vi "SetFunctionClass.vi"(8 "error in (no error)":errorcluster, 10 "FunctionClass":variant, 11 "AnalysisPluginsBase in":refnum<class "AnalysisPluginsBase.lvclass">) -> (0 "error out":errorcluster, 3 "AnalysisPluginsBase out":refnum<class "AnalysisPluginsBase.lvclass">)   [LabVIEW 2018, in "AnalysisPlugins.lvlib" / "AnalysisPluginsBase.lvclass"]
uses:
  AnalysisPluginsBase.lvclass
  <userlib>/NIST/BaseClasses/Object_class/BaseObject.lvclass
panel:
  # "Not all analysis plugins will\nhave function classes"
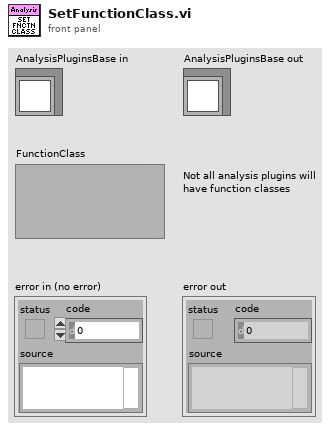
[diagram p1: front panel]
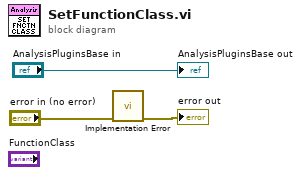
[diagram p0: block diagram]
diagram:
  n1 = call <userlib>:"Implementation Error.vi"("error in (no error)"="error in (no error)") -> ("error out"=→"error out":errorcluster)  [unwired: 10 in]
  "AnalysisPluginsBase out" <- "AnalysisPluginsBase in"
